vi "First.vi"(8 "error in (no error)":errorcluster) -> (0 "error out":errorcluster, 3 "Quem começa":bool)   [LabVIEW 2017]
doc: "SubVI criada para que o usuário escolha quem começa em caso de partida contra o computador"
panel:
  in  "PC":bool
  in  "Player":bool
  # "Quem começa?"
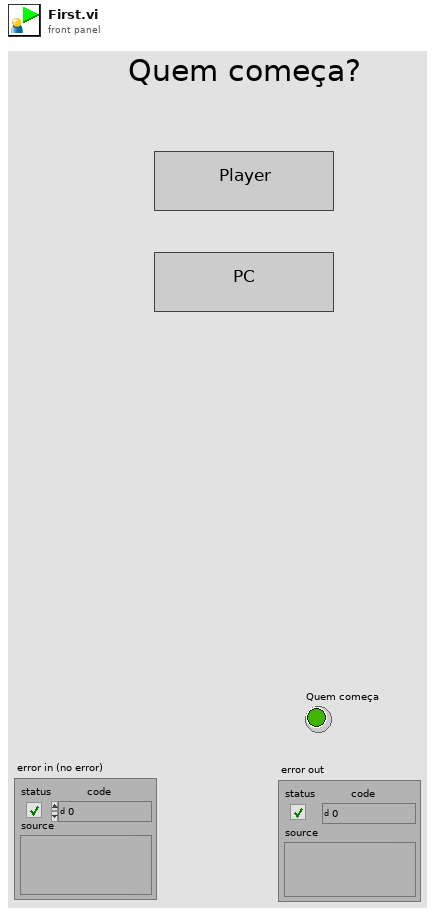
[diagram p1: front panel]
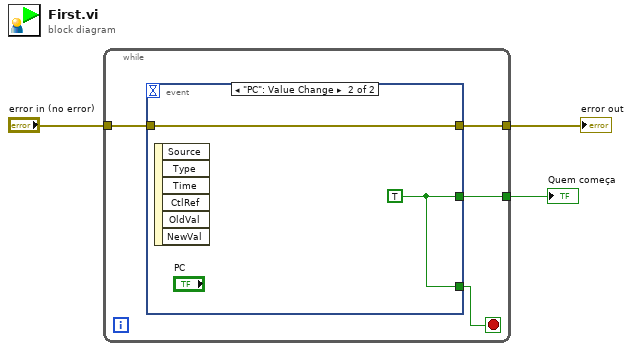
[diagram p0: block diagram]
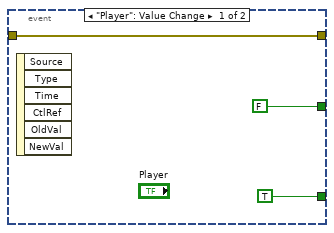
[diagram p2: hidden frame]
diagram:
  n1 = while {
    tunnel: [w6] -> w3
    tunnel: "error in (no error)" -> [w5]
    tunnel: [w4] -> w1
    stop <- w7 stop-if-true
    n2 = event shown="[1] \"PC\": Value Change" {
      selector: _ -> [_ _]
      dyn-events: _ -> [_ _]
      timeout: _ -> [_ _]
      tunnel: [TRUE w12] -> w7
      tunnel: [FALSE w12] -> w6
      tunnel: w5 -> [w8 w11]
      tunnel: [w8 w11] -> w4
      event "Player": Value Change {
        n3 = event-data() -> ()  [unwired: 1 in, 6 out]
      }
      event "PC": Value Change {
        w12 = TRUE
        n4 = event-data() -> ()  [unwired: 1 in, 6 out]
      }
    }
  }
  "Quem começa" <- w3
  "error out" <- w1
